vi "GE 5565PIORC.DMA.Block.Read (DBL).vi"(8 "error in (no error)":errorcluster, 9 "count":u32, 10 "Block Descriptor in":T1 {"descriptor params"."data ptr (lower)" format="%.0x"; "descriptor params"."data ptr (upper)" format="%.0x"; "descriptor params"."data size" format="%.0x"; "descriptor params"."next descriptor ptr" format="%.0x"; "descriptor size" format="%08x"; "descriptor ptr (RFM)" format="%08x"; "descriptor ptr (VISA)" format="%08x"}, 11 "GE 5565PIORC in":refnum<class "GE 5565PIORC.lvclass">) -> (0 "error out":errorcluster, 1 "data out":dbl[](array[numeric]), 2 "Block Descriptor out":T1 {"descriptor params"."data ptr (lower)" format="%.0x"; "descriptor params"."data ptr (upper)" format="%.0x"; "descriptor params"."data size" format="%.0x"; "descriptor params"."next descriptor ptr" format="%.0x"; "descriptor size" format="%08x"; "descriptor ptr (RFM)" format="%08x"; "descriptor ptr (VISA)" format="%08x"}, 3 "GE 5565PIORC out":refnum<class "GE 5565PIORC.lvclass">)   [LabVIEW 2016, in "GE 5565PIORC.lvclass"]
doc: "Reads <B>count</B> elements from the provided <B>Block Descriptor</B> into a newly allocated <B>data</B> array."
uses:
  GE 5565PIORC.lvclass
  Typedefs/GE 5565PIORC.Typedef.DMA Block Descriptor.ctl
  Typedefs/GE 5565PIORC.Typedef.DMA Block Descriptor Params.ctl
  <vilib>/Instr/_visa.llb/VISA Register Access Address Space.ctl
  GE 5565PIORC.lvclass/GE 5565PIORC.ctl
  GE 5565PIORC.VISA.Move In.String (U8).vi
  GE 5565PIORC.VISA.Return Handler.vi
  <vilib>/Utility/error.llb/Error Cluster From Error Code.vi
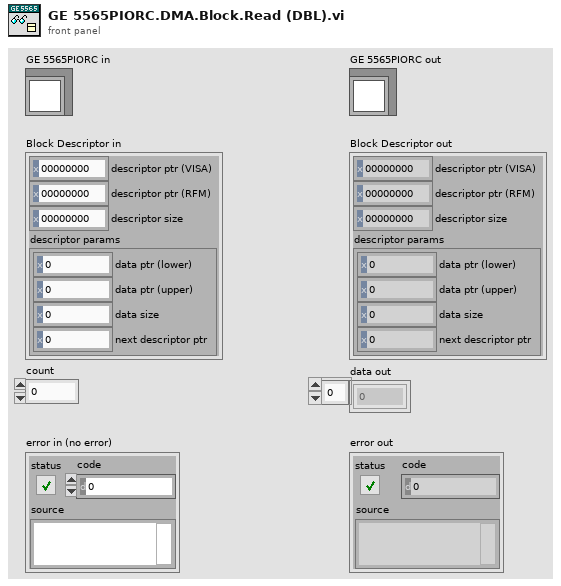
[diagram p1: front panel]
types:
  T1 = typedef "GE 5565PIORC.lvclass/GE 5565PIORC.Typedef.DMA Block Descriptor.ctl" = cluster{"descriptor ptr (VISA)":u32, "descriptor ptr (RFM)":u32, "descriptor size":u32, "descriptor params":T2}
  T2 = typedef "GE 5565PIORC.lvclass/GE 5565PIORC.Typedef.DMA Block Descriptor Params.ctl" = cluster{"data ptr (lower)":u32, "data ptr (upper)":u32, "data size":u32, "next descriptor ptr":u32}
  T3 = typedef "VISA Register Access Address Space.ctl" = u16
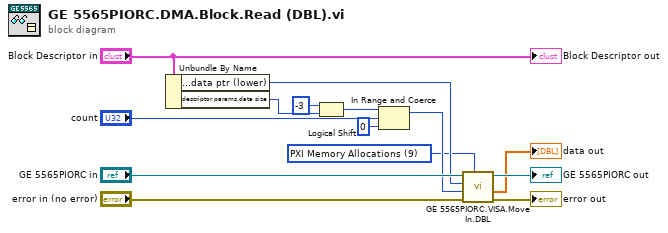
[diagram p0: block diagram]
diagram:
  w2 = T3 9 items=["VXI/VME A16"=1, "VXI/VME A24"=2, "VXI/VME A32"=3, "VXI/VME A64"=4, "PXI Memory Allocations"=9, "PXI Configuration"=10, "PXI BAR0"=11, "PXI BAR1"=12, "PXI BAR2"=13, "PXI BAR3"=14, "PXI BAR4"=15, "PXI BAR5"=16] ("address space")
  n1 = Unbundle By Name("Block Descriptor in") -> ("descriptor params.data ptr (lower)"=w4:u32, "descriptor params.data size"=w5:u32)
  n2 = Logical Shift(y=i16 -3, x=w5) -> (x << y=w10:u32)
  n3 = In Range and Coerce(upper limit=w10, x="count", lower limit=u32 0) -> (coerced(x)=w3:u32)  [unwired: 1 out]
  n4 = call "GE 5565PIORC.VISA.Move In.DBL.vi"("address space"=w2, "error in (no error)"="error in (no error)", "count"=w3, "offset"=w4, "GE 5565PIORC in"="GE 5565PIORC in") -> ("error out"=→"error out":errorcluster, "data out"=→"data out":dbl[], "GE 5565PIORC out"=→"GE 5565PIORC out":refnum<class "GE 5565PIORC.lvclass">)  [unwired: 4 in]
  "Block Descriptor out" <- "Block Descriptor in"
